vi "Measurement Logic.vi"() -> ()   [LabVIEW 2021, in "Efficiency And Load Regulation with Pin Map.lvlib"]
uses:
  Efficiency And Load Regulation with Pin Map.lvlib
  Measurement Configuration.ctl
  <instrlib>/niScope/Controls/niScope vertical coupling.ctl
  <instrlib>/niDMM/nidmm.llb/niDMM Resolution in Digits.ctl
  Measurement Results.ctl
  <vilib>/Plug-In SDKs/Measurements/Measure Call Context/Measure Call Context.lvclass
  subVIs/Reference values.ctl
  <vilib>/Plug-In SDKs/Clients/Session Management V1/Session Reservation/Session Reservation.lvclass
  common/Instrument Control/Scope/TClk/Instrument Info.ctl
  common/Instrument Control/Scope Parameters.ctl
  <instrlib>/niDMM/nidmm.llb/niDMM Trigger.ctl
  <instrlib>/niDMM/nidmm.llb/niDMM Sample Trigger.ctl
  subVIs/Additional measurements.ctl
  common/Instrument Control/DCPower Parameters.ctl
  <vilib>/Plug-In SDKs/Measurements/Measure Call Context/Reserve Sessions - NPin.vi
  <vilib>/Plug-In SDKs/Sessions/niDCPower/Initialize Sessions - NSess.vi
  <vilib>/Plug-In SDKs/Sessions/niDCPower/Get Connections - NPin MConn.vi
  <vilib>/Plug-In SDKs/Sessions/niDCPower/Get Connections - 1Pin 1Conn.vi
  <vilib>/Plug-In SDKs/Sessions/niScope/Initialize Sessions - NSess.vi
  <vilib>/Plug-In SDKs/Sessions/niScope/Get Connections - NPin MConn.vi
  <instrlib>/niScope/Configure/Trigger/niScope Configure Trigger Digital.vi
  <vilib>/Plug-In SDKs/Sessions/niDMM/Initialize Sessions - NSess.vi
  <vilib>/Plug-In SDKs/Sessions/niDMM/Get Connections - NPin MConn.vi
  <vilib>/Plug-In SDKs/Sessions/niDCPower/NI Session Management niDCPower.lvlib
  <vilib>/Plug-In SDKs/Sessions/niScope/NI Session Management niScope.lvlib
  common/PMIC Common.lvlib
  <vilib>/Plug-In SDKs/Sessions/niDMM/NI Session Management niDMM.lvlib
panel:
  out "measure call context out":refnum<class "Measure Call Context.lvclass">
  in  "measure call context in":refnum<class "Measure Call Context.lvclass">
  out "measurement results":T1
  in  "measurement configuration":T2={"Mode of operation"=enum."Perform measurement", "DUT setup time"=1.0, "Source delay"=0.005, "Aperture time"=0.005, "Nominal output voltage"=3.3, "Source pin name array"=[], "Source pin name index for efficiency"=0, "Source sense array"=[], "Source current limit array"=[], "Source maximum power array"=[], "Source start voltage array"=[], "Source stop voltage array"=[], "Source voltage sweep points"=10, "Use Source voltage array"=FALSE, "Source voltage concatenated array"=[], "Source voltage array size"=[], "Load pin name"="", "Load sense"=1009, "Load voltage limit range"=6.0, "Load sweep type"="Logarithmic", "Load start current"=0.1, "Load stop current"=24.0, "Load current sweep points/points per decade"=10, "Use Load current array"=FALSE, "Load current array"=[], "Pin Names for Scope"=[], "vertical range"=[], "vertical offset"=[], "probe attenuation"=[], "vertical coupling"=[], "channel enabled"=[], "input impedance"=[], "max input frequency"=[], "min sample rate"=[], "reference position"=[], "min record length"=[], "enforce realtime"=[], "dmm pin names"=[], "dmm function array"=[], "dmm resolution in digits array"=[], "dmm range array"=[]} {"dmm function array" items=["DC Volts", "AC Volts", "DC Current", "AC Current", "2-wire Resistance", "4-wire Resistance", "Diode", "Frequency", "Period", "AC Volts DC Coupled", "Capacitance", "Inductance", "Temperature"]; "Source sense array" items=["Local"=1008, "Remote"=1009]; "dmm resolution in digits array" items=["3 1/2"=3.5, "4 1/2"=4.5, "5 1/2"=5.5, "6 1/2"=6.5, "7 1/2"=7.5]; "input impedance" items=["1 mega ohm"=0, "50 ohms"=2]; "vertical coupling" items=["AC", "DC", "Ground"]; "Load sense" items=["Local"=1008, "Remote"=1009]}
  out "error out":errorcluster
  in  "error in":errorcluster
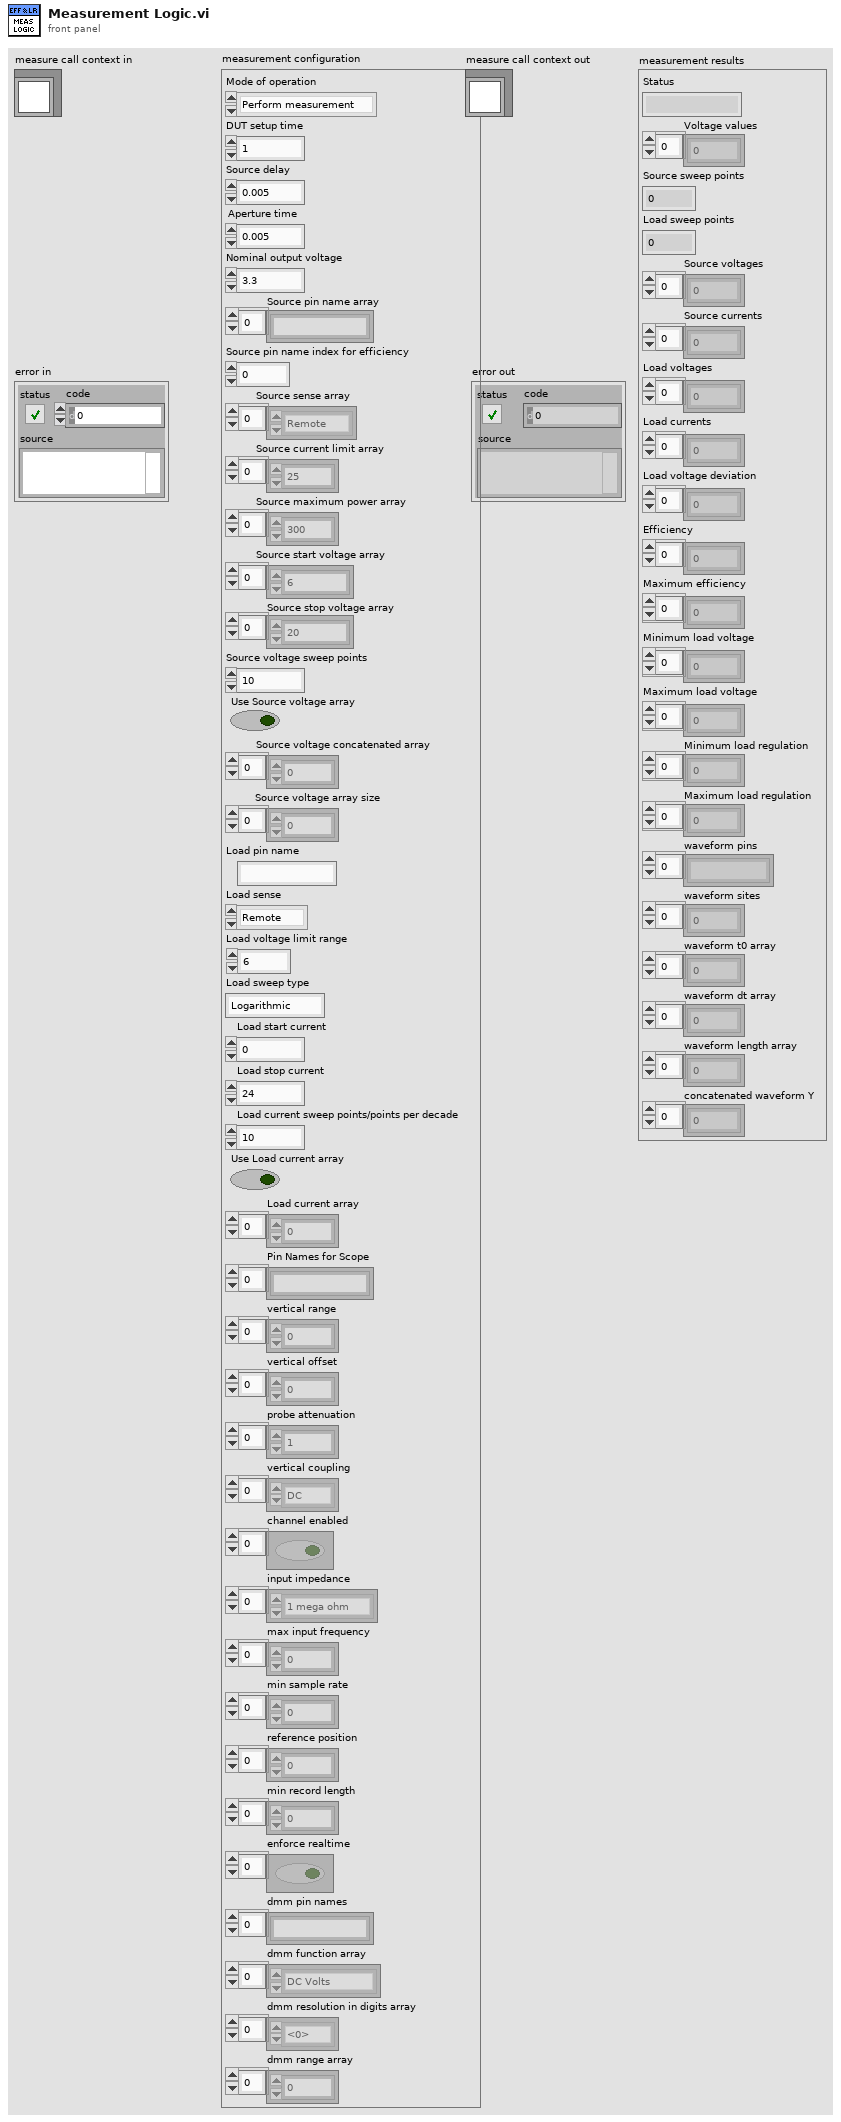
[diagram p1: front panel]
types:
  T1 = typedef "Efficiency And Load Regulation with Pin Map.lvlib/Measurement Results.ctl" = cluster{"Status":string, "Voltage values":dbl[], "Source sweep points":i32, "Load sweep points":i32, "Source voltages":dbl[], "Source currents":dbl[], "Load voltages":dbl[], "Load currents":dbl[], "Load voltage deviation":dbl[], "Efficiency":dbl[], "Maximum efficiency":dbl[], "Minimum load voltage":dbl[], "Maximum load voltage":dbl[], "Minimum load regulation":dbl[], "Maximum load regulation":dbl[], "waveform pins":string[], "waveform sites":i32[], "waveform t0 array":dbl[], "waveform dt array":dbl[], "waveform length array":i32[], "concatenated waveform Y":dbl[]}
  T2 = typedef "Efficiency And Load Regulation with Pin Map.lvlib/Measurement Configuration.ctl" = cluster{"Mode of operation":enum32{"Power on the DUT", "Perform measurement", "Power off the DUT"}, "DUT setup time":dbl, "Source delay":dbl, "Aperture time":dbl, "Nominal output voltage":dbl, "Source pin name array":string[], "Source pin name index for efficiency":i32, "Source sense array":i32[], "Source current limit array":dbl[], "Source maximum power array":dbl[], "Source start voltage array":dbl[], "Source stop voltage array":dbl[], "Source voltage sweep points":i32, "Use Source voltage array":bool, "Source voltage concatenated array":dbl[], "Source voltage array size":i32[], "Load pin name":string, "Load sense":i32, "Load voltage limit range":dbl, "Load sweep type":string, "Load start current":dbl, "Load stop current":dbl, "Load current sweep points/points per decade":i32, "Use Load current array":bool, "Load current array":dbl[], "Pin Names for Scope":string[], "vertical range":dbl[], "vertical offset":dbl[], "probe attenuation":dbl[], "vertical coupling":T3[], "channel enabled":bool[], "input impedance":u32[], "max input frequency":dbl[], "min sample rate":dbl[], "reference position":dbl[], "min record length":i32[], "enforce realtime":bool[], "dmm pin names":string[], "dmm function array":u32[], "dmm resolution in digits array":T4[], "dmm range array":dbl[]}
  T3 = typedef "niScope vertical coupling.ctl" = i32
  T4 = typedef "niDMM Resolution in Digits.ctl" = dbl
  T5 = typedef "Efficiency And Load Regulation with Pin Map.lvlib/Reference values.ctl" = cluster{"dcpower session reservation":refnum<class "Session Reservation.lvclass">, "Source handle array":refnum<k15>[], "Source channel name array":string[], "Load handle":refnum<k15>, "Load channel name":string, "Source voltage values":dbl[][], "Load current values":dbl[], "Number of steps":i32, "Source sequence name":string, "Source terminal name":string, "Measure terminal name":string, "scope session reservation":refnum<class "Session Reservation.lvclass">, "Scope handles":refnum<k15>[][], "connection map":map{string, T6[]}, "instrument info map array":map{string, cluster{"channel":string, "siteNumber":i32, "pin":string, "Scope Parameters":T7}[]}[], "Enable TClk":bool, "dmm session reservation":refnum<class "Session Reservation.lvclass">, "dmm handle array":refnum<k15>[], "DMM Trigger Source":T8, "DMM Sample Trigger":T9, "Measurement Results":T1, "Additional measurements":T10}
  T6 = typedef "PMIC Common.lvlib/Instrument Info.ctl" = cluster{"instrument":string, "channel":string, "siteNumber":i32}
  T7 = typedef "PMIC Common.lvlib/Scope Parameters.ctl" = cluster{"vertical range":dbl, "vertical offset":dbl, "probe attenuation":dbl, "vertical coupling":T3, "channel enabled":bool, "input impedance":u32, "maximum input frequency":dbl, "min sample rate":dbl, "reference position":dbl, "min record length":i32, "number of records":i32, "enforce realtime":bool}
  T8 = typedef "niDMM Trigger.ctl" = enum16{"Immediate", "External", "TTL 0", "TTL 1", "TTL 2", "TTL 3", "TTL 4", "TTL 5", "TTL 6", "Software", "TTL 7", "PXI Star", "LBR Trig 1", "Aux Trig 1"}
  T9 = typedef "niDMM Sample Trigger.ctl" = enum16{"Immediate", "External", "TTL 0", "TTL 1", "TTL 2", "TTL 3", "TTL 4", "TTL 5", "TTL 6", "Interval", "Software", "TTL 7", "PXI Star", "LBR Trig 1", "Aux Trig 1"}
  T10 = typedef "Efficiency And Load Regulation with Pin Map.lvlib/Additional measurements.ctl" = cluster{"voltage measurements from all sources":dbl[][], "current measurements from all sources":dbl[][], "all dmm measurements":dbl[][], "all scope waverforms":waveform(dbl)[]}
  T11 = enum32{"Power on the DUT", "Perform measurement", "Power off the DUT"}
  T12 = typedef "PMIC Common.lvlib/DCPower Parameters.ctl" = cluster{"Supply":dbl, "Limit":dbl, "Aperture Time":dbl, "Settling Time":dbl, "Sense":i32, "Transient Response":i32}
  T13 = enum16{"PXI_Trig0", "PXI_Trig1", "PXI_Trig2", "PXI_Trig3", "PXI_Trig4", "PXI_Trig5", "PXI_Trig6", "PXI_Trig7"}
  T14 = typedef "NI Session Management niDCPower.lvlib/Connection with Session.ctl" = cluster{"connection":T15, "session":refnum<k15>}
  T15 = typedef "NI Session Management V1 Client.lvlib/Session Reservation.lvclass/Connection.ctl" = cluster{"pin or relay name":string, "site":i32, "instrument type id":string, "channel":string}
  T16 = typedef "PMIC Common.lvlib/DCPower Parameters for Adv Sequence.ctl" = cluster{"Supplies":dbl[], "Limits":dbl[], "Aperture Time":dbl, "Settling Time":dbl, "Sense":i32, "Transient Response":i32}
  T17 = typedef "PMIC Common.lvlib/DCPower Parameters for Sequence.ctl" = cluster{"Supplies":dbl[], "Limit":dbl, "Aperture Time":dbl, "Settling Time":dbl, "Sense":i32, "Transient Response":i32}
  T18 = typedef "NI Session Management niScope.lvlib/Connection with Session.ctl" = cluster{"connection":T15, "session":refnum<k15>}
  T19 = typedef "NI Measurement Plug-In SDK.lvlib/Pin Map Context.ctl" = cluster{"pin map id":string, "sites":i32[]}
  T20 = map{string, cluster{"channel":string, "siteNumber":i32, "pin":string, "Scope Parameters":T7}[]}[]
  T21 = typedef "NI Session Management niDMM.lvlib/Connection with Session.ctl" = cluster{"connection":T15, "session":refnum<k15>}
  T22 = typedef "PMIC Common.lvlib/DMM Parameters.ctl" = cluster{"Function":T23, "Resolution in Digits":T4, "Range":dbl, "Trigger Source":T8, "Trigger Delay (sec)":dbl, "Trigger Count":i32, "Sample Count":i32, "Sample Trigger":T9, "Sample Interval (sec)":dbl, "Trigger Slope":T24, "Sample Trigger Slope":T24}
  T23 = typedef "niDMM Function.ctl" = enum16{"DC Volts", "AC Volts", "DC Current", "AC Current", "2-wire Resistance", "4-wire Resistance", "Diode", "Frequency", "Period", "AC Volts DC Coupled", "Capacitance", "Inductance", "Temperature"}
  T24 = typedef "niDMM Slope.ctl" = enum16{"Rising Edge", "Falling Edge"}
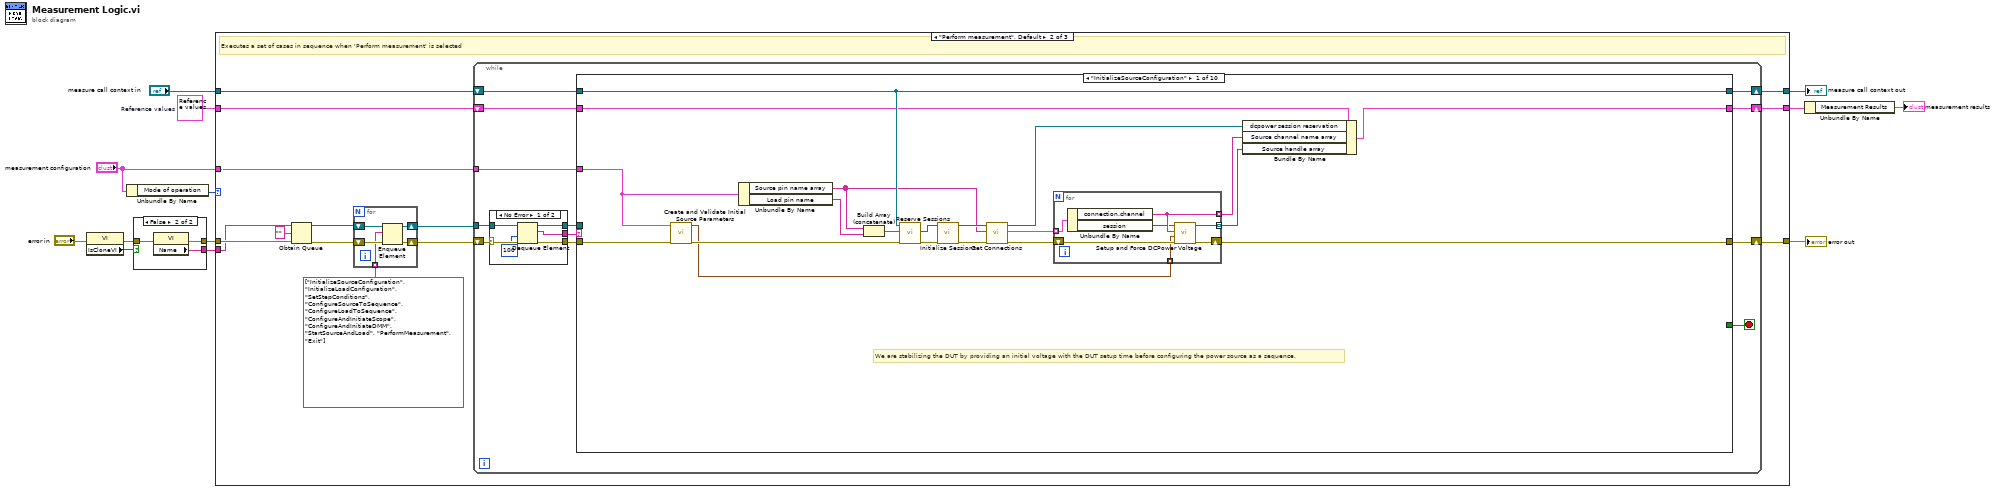
[diagram p0: block diagram]
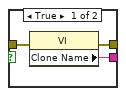
[diagram p2: hidden frame]
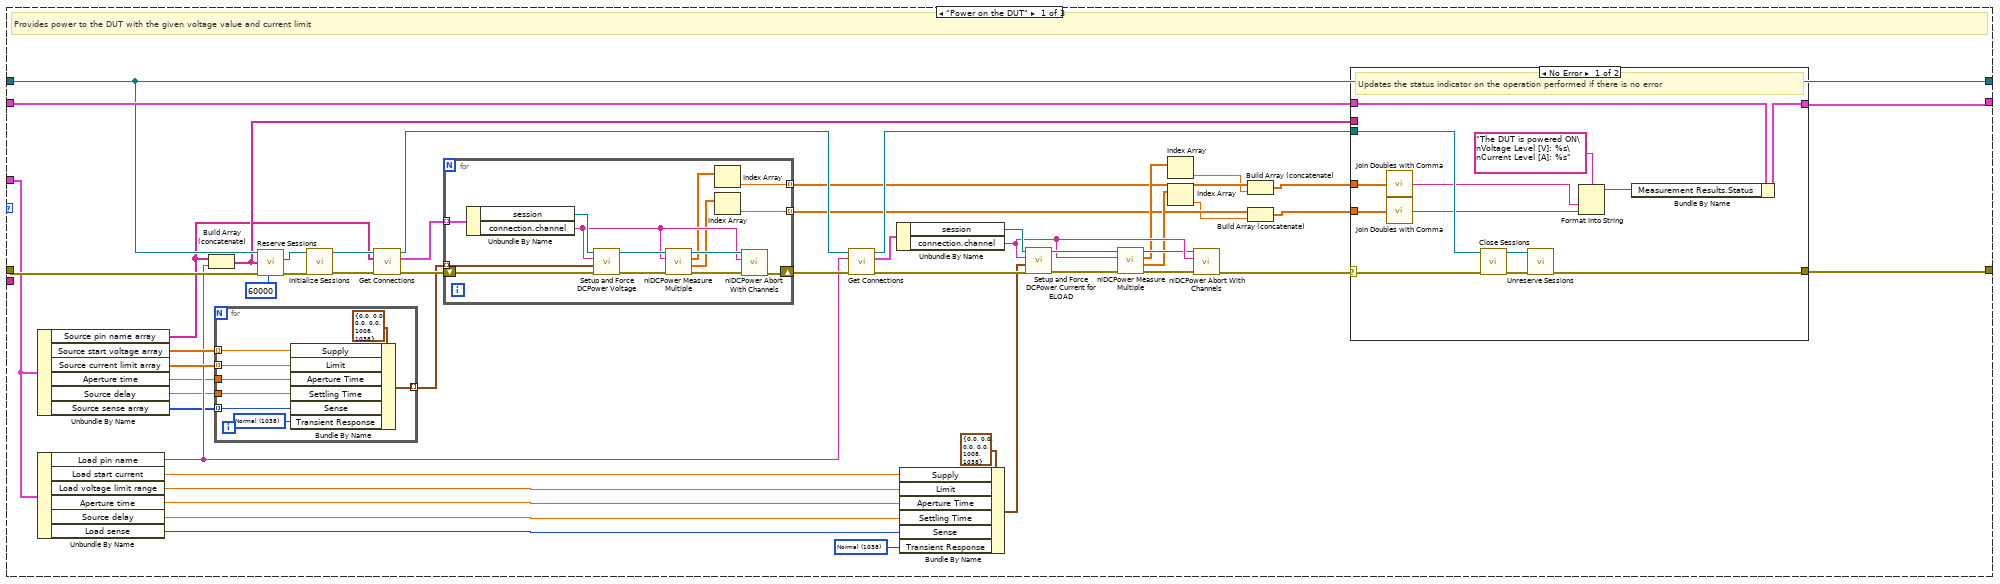
[diagram p3: hidden frame]
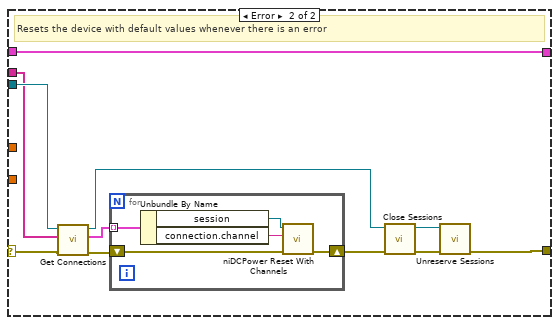
[diagram p4: hidden frame]
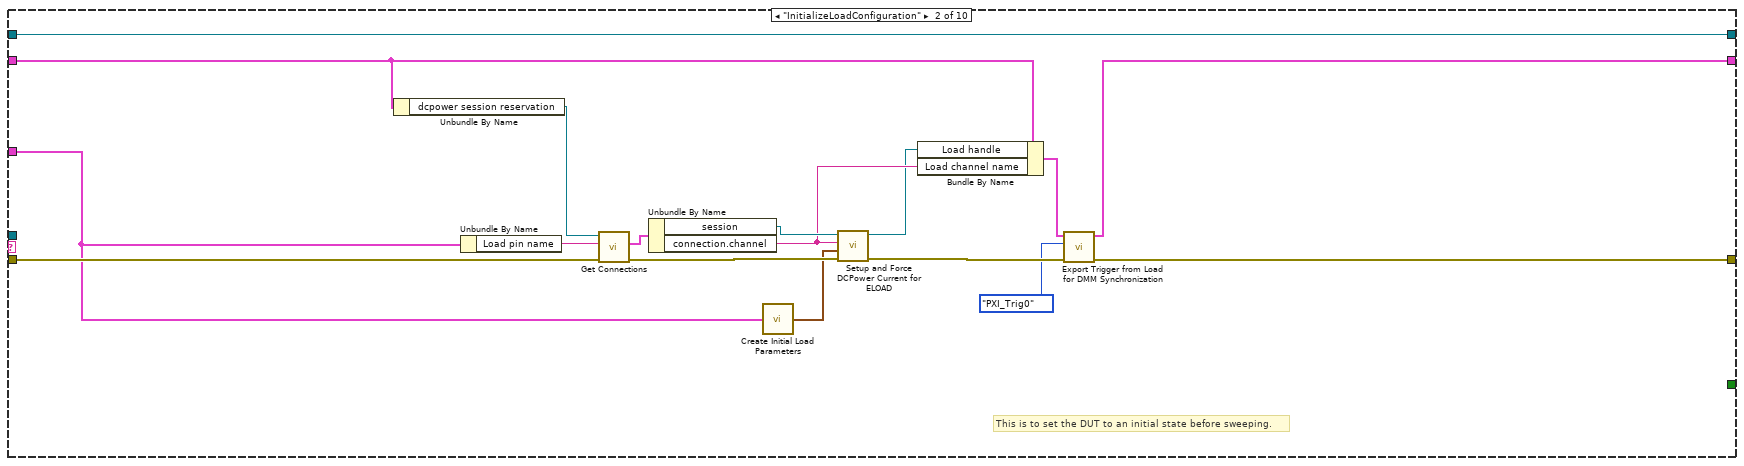
[diagram p5: hidden frame]
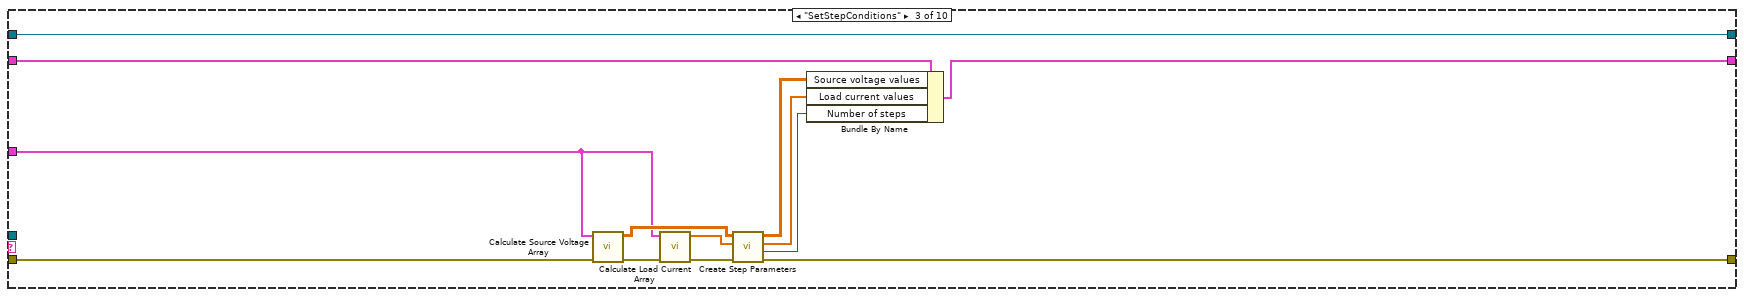
[diagram p6: hidden frame]
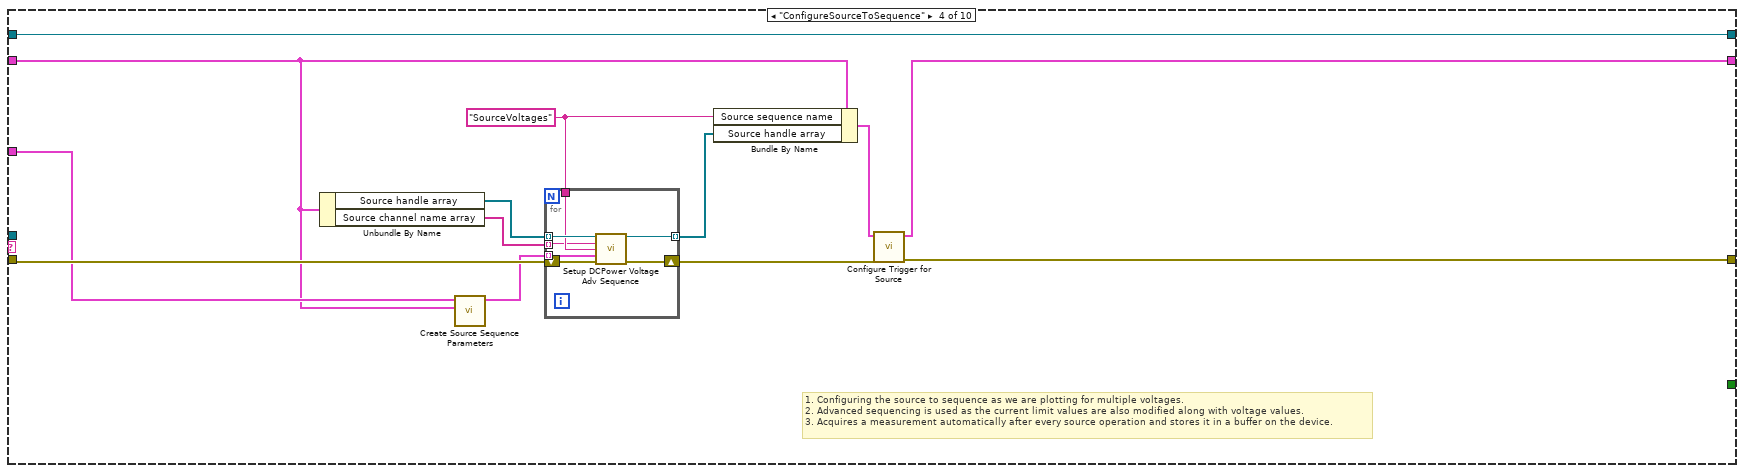
[diagram p7: hidden frame]
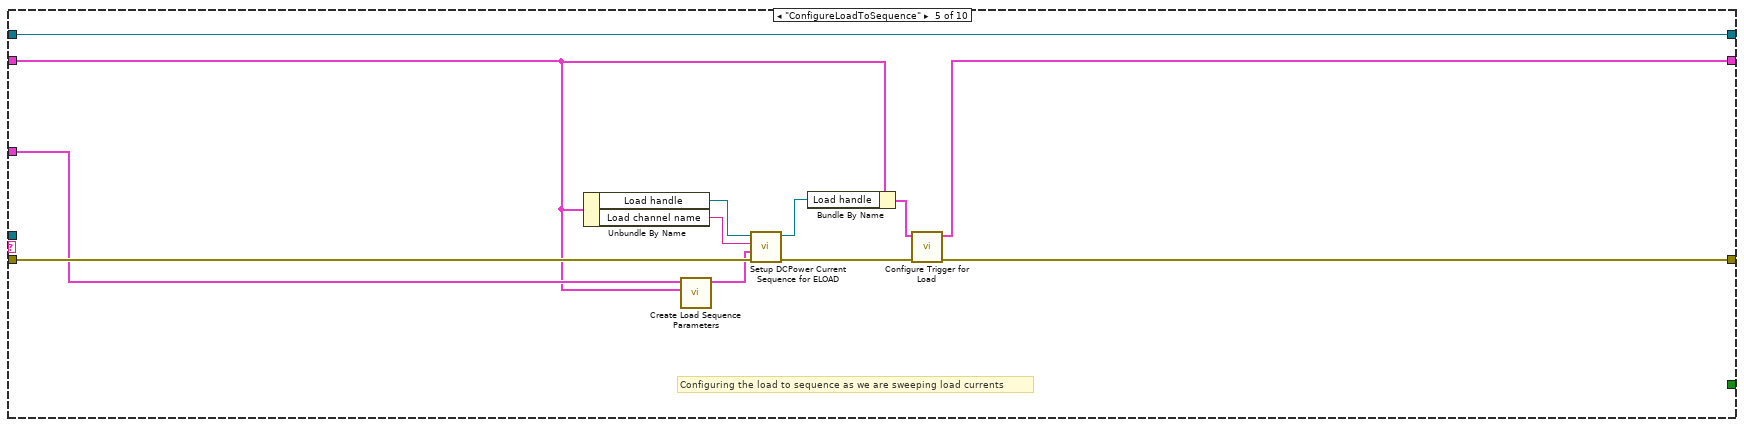
[diagram p8: hidden frame]
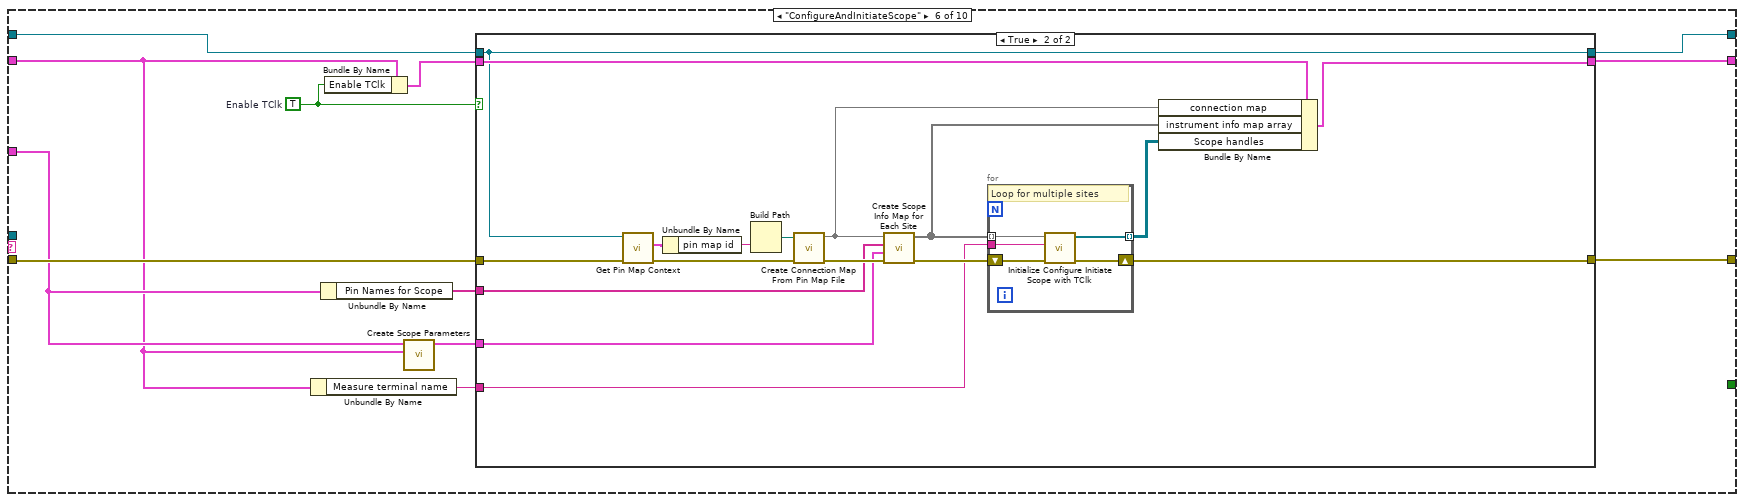
[diagram p9: hidden frame]
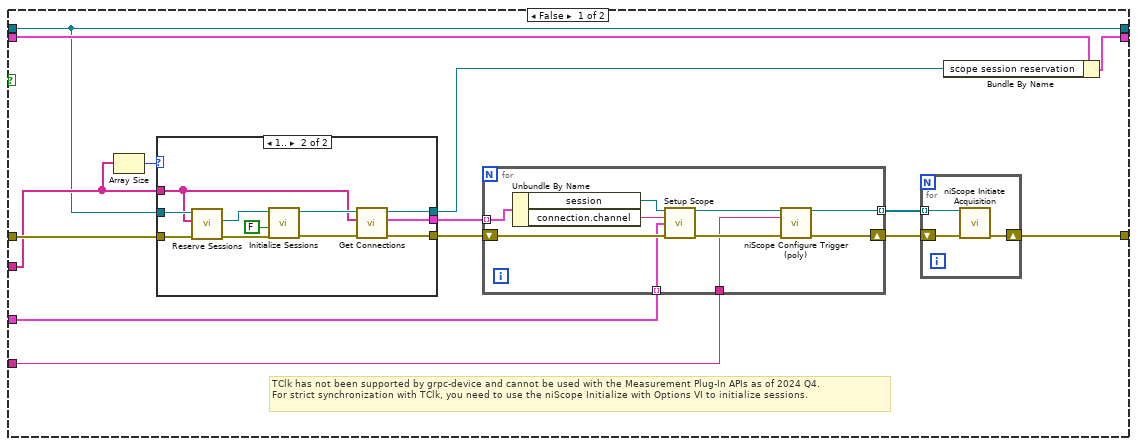
[diagram p10: hidden frame]
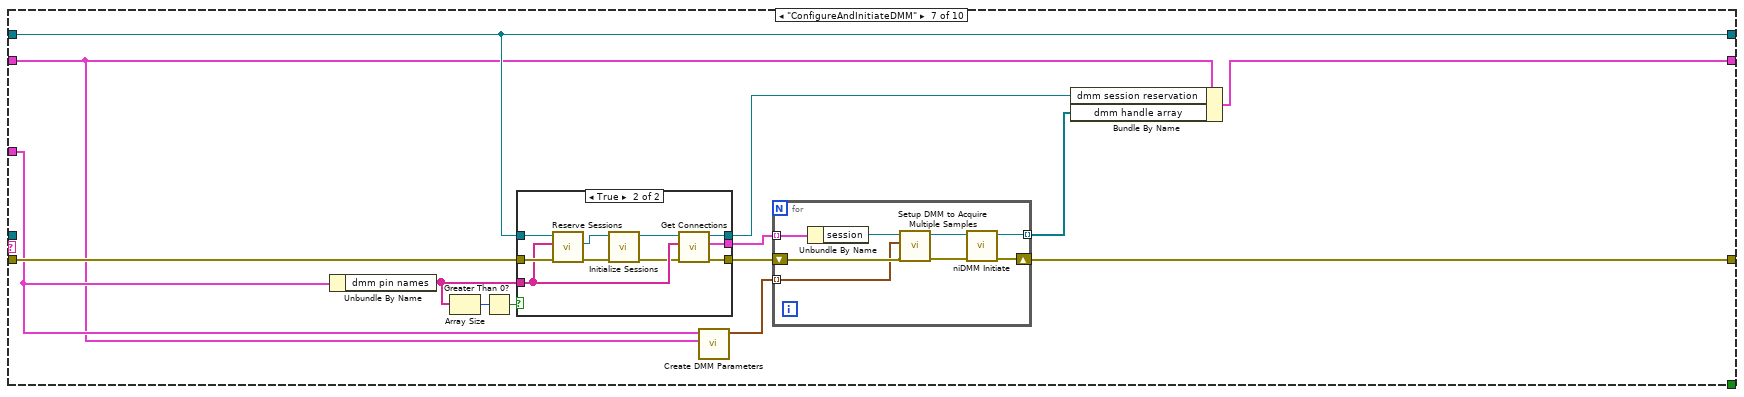
[diagram p12: hidden frame]
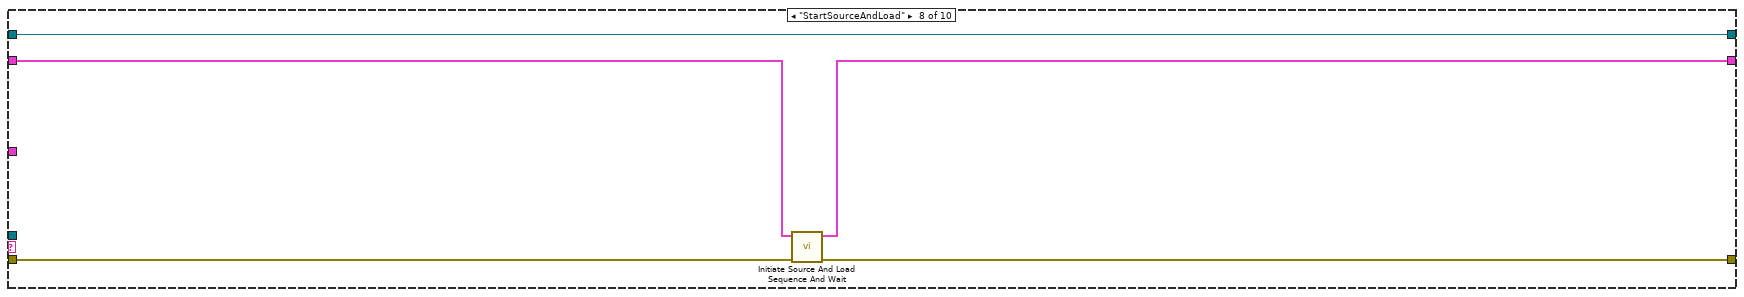
[diagram p14: hidden frame]
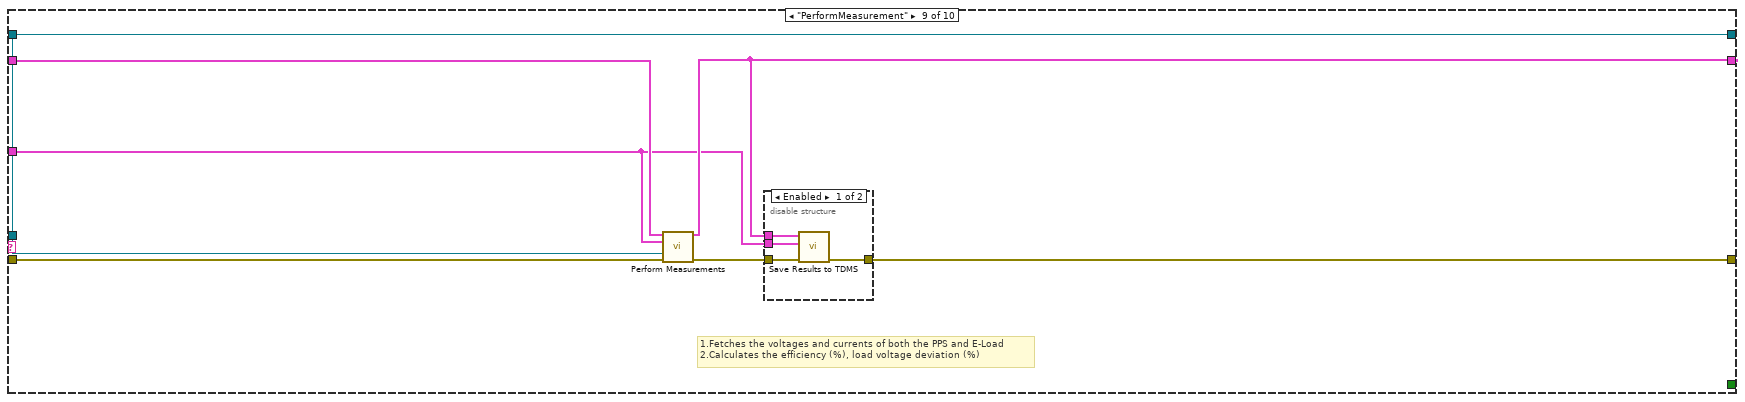
[diagram p15: hidden frame]
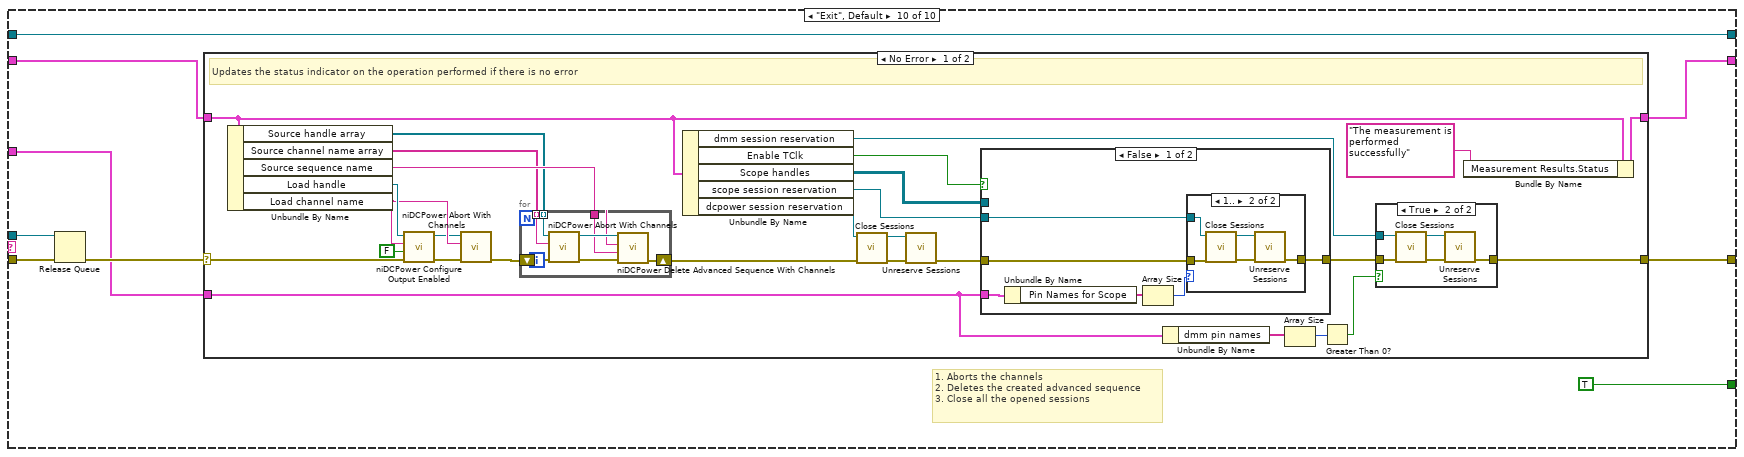
[diagram p17: hidden frame]
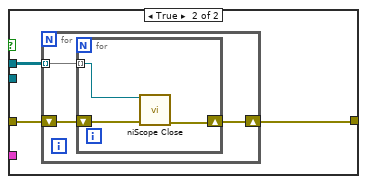
[diagram p20: hidden frame]
diagram:
  w12 = T5 {"dcpower session reservation"=refnum, "Source handle array"=[], "Source channel name array"=[], "Load handle"="", "Load channel name"="", "Source voltage values"=[], "Load current values"=[], "Number of steps"=0, "Source sequence name"="", "Source terminal name"="", "Measure terminal name"="", "scope session reservation"=refnum, "Scope handles"=[], "connection map"={}, "instrument info map array"=[], "Enable TClk"=FALSE, "dmm session reservation"=refnum, "dmm handle array"=[], "DMM Trigger Source"=enum."Immediate", "DMM Sample Trigger"=enum."TTL 0", "Measurement Results"={"Status"="", "Voltage values"=[], "Source sweep points"=0, "Load sweep points"=0, "Source voltages"=[], "Source currents"=[], "Load voltages"=[], "Load currents"=[], "Load voltage deviation"=[], "Efficiency"=[], "Maximum efficiency"=[], "Minimum load voltage"=[], "Maximum load voltage"=[], "Minimum load regulation"=[], "Maximum load regulation"=[], "waveform pins"=[], "waveform sites"=[], "waveform t0 array"=[], "waveform dt array"=[], "waveform length array"=[], "concatenated waveform Y"=[]}, "Additional measurements"={"voltage measurements from all sources"=[], "current measurements from all sources"=[], "all dmm measurements"=[], "all scope waverforms"=[]}}  # Reference values
  n1 = property class="VI"(error in="error in") -> (error out=w4:errorcluster, "IsCloneVI"=w5:bool)  [unwired: 1 in, 1 out]
  n2 = Unbundle By Name("measurement configuration") -> ("Mode of operation"=w10:T11)
  n3 = case shown="False" w5 {
    tunnel: [w16 w19] -> w2
    tunnel: [w15 w18] -> w1
    tunnel: w4 -> [w14 w17]
    frame True {
      n4 = property class="VI"(error in=w14) -> (error out=w16:errorcluster, "Clone Name"=w15:string)  [unwired: 1 in, 1 out]
    }
    frame False {
      n5 = property class="VI"(error in=w17) -> (error out=w19:errorcluster, "Name"=w18:string)  [unwired: 1 in, 1 out]
    }
  }
  n6 = case shown="\"Perform measurement\", Default" w10 {
    tunnel: [w67 w122 w502] -> w6
    tunnel: w2 -> [w57 w123 w521]
    tunnel: "measurement configuration" -> [w31 w129 w530]
    tunnel: [w68 w124 w527] -> w7
    tunnel: w12 -> [w69 w128 w529]
    tunnel: "measure call context in" -> [w58 w126 w519]
    tunnel: [w58 w125 w519] -> w8
    tunnel: w1 -> [_ w121 _]
    frame "Power on the DUT" {
      w22 = 1038 items=["Slow"=1041, "Normal"=1038, "Fast"=1039, "Custom"=1042] ("Transient Response")
      # "Provides power to the DUT with the given voltage value and current limit"
      n7 = Unbundle By Name(w31) -> ("Source pin name array"=w32:string[], "Source start voltage array"=w60:dbl[], "Source current limit array"=w59:dbl[], "Aperture time"=w28:dbl, "Source delay"=w27:dbl, "Source sense array"=w26:i32[])
      n8 = Unbundle By Name(w31) -> ("Load pin name"=w30:string, "Load start current"=w25:dbl, "Load voltage limit range"=w24:dbl, "Aperture time"=w21:dbl, "Source delay"=w20:dbl, "Load sense"=w23:i32)
      n9 = Build Array (concatenate)(w32, w30) -> (w33:string[])
      n10 = for {
        tunnel: w60 -> [w77] mode=indexing
        tunnel: w59 -> [w76] mode=indexing
        tunnel: [w74] -> w29 mode=indexing
        tunnel: w28 -> [w73]
        tunnel: w27 -> [w71]
        tunnel: w26 -> [w72] mode=indexing
        w70 = 1038 items=["Slow"=1041, "Normal"=1038, "Fast"=1039, "Custom"=1042] ("Transient Response")
        n11 = Bundle By Name(cluster=T12 {"Supply"=0.0, "Limit"=0.0, "Aperture Time"=0.0, "Settling Time"=0.0, "Sense"=1008, "Transient Response"=1038} ("DCPower Parameters"), "Supply"=w77, "Limit"=w76, "Aperture Time"=w73, "Settling Time"=w71, "Sense"=w72, "Transient Response"=w70) -> (w74:T12)
      }
      n12 = call-poly <vilib>:"Reserve Sessions.vi"("timeout (ms)"=60000, "error in"=w57, "pin or relay names"=w33, "measurement context in"=w58) -> ("error out"=w66:errorcluster, "session reservation out"=w65:refnum<class "Session Reservation.lvclass">)  [unwired: 5 in, 1 out]
      n13 = call-poly <vilib>:"Initialize Sessions.vi"("error in"=w66, "session reservation in"=w65) -> ("error out"=w64:errorcluster, "session reservation out"=w63:refnum<class "Session Reservation.lvclass">)  [unwired: 6 in, 2 out]
      n14 = call-poly <vilib>:"Get Connections.vi"("error in"=w64, "pin or relay names"=w32, "session reservation in"=w63) -> ("error out"=w61:errorcluster, "connections"=w56:T14[], "session reservation out"=w53:refnum<class "Session Reservation.lvclass">)  [unwired: 6 in]
      n15 = for {
        tunnel: w56 -> [w90] mode=indexing
        tunnel: w29 -> [w88] mode=indexing
        shift-right: [w85] -> w55
        shift-left: w61 -> [w91]
        tunnel: [w79] -> w39 mode=indexing
        tunnel: [w78] -> w36 mode=indexing
        n16 = Unbundle By Name(w90) -> ("session"=w89:refnum<k15>, "connection.channel"=w82:string)
        n17 = call "Setup and Force DCPower Voltage.vi"("error in"=w91, "Parameters"=w88, "Channel List"=w82, "DCPower Handle In"=w89) -> ("error out"=w87:errorcluster, "DCPower Handle Out"=w86:refnum<k15>)  [unwired: 6 in]
        n18 = call <instrlib>:"niDCPower Measure Multiple.vi"("error in (no error)"=w87, "channel name"=w82, "instrument handle"=w86) -> ("error out"=w84:errorcluster, "current measurements"=w80:dbl[], "voltage measurements"=w81:dbl[], "instrument handle out"=w83:refnum<k15>)  [unwired: 5 in]
        n19 = Index Array(array=w81) -> (element=w79:dbl)  [unwired: 1 in]
        n20 = Index Array(array=w80) -> (element=w78:dbl)  [unwired: 1 in]
        n21 = call <instrlib>:"niDCPower Abort With Channels.vi"("error in (no error)"=w84, "channel name"=w82, "instrument handle"=w83) -> ("error out"=w85:errorcluster)  [unwired: 7 in, 1 out]
      }
      n22 = call-poly <vilib>:"Get Connections.vi"("error in"=w55, "pin or relay name"=w30, "session reservation in"=w53) -> ("error out"=w50:errorcluster, "connection"=w54:T14, "session reservation out"=w52:refnum<class "Session Reservation.lvclass">)  [unwired: 6 in]
      n23 = Unbundle By Name(w54) -> ("session"=w51:refnum<k15>, "connection.channel"=w43:string)
      n24 = Bundle By Name(cluster=T12 {"Supply"=0.0, "Limit"=0.0, "Aperture Time"=0.0, "Settling Time"=0.0, "Sense"=1008, "Transient Response"=1038} ("DCPower Parameters"), "Supply"=w25, "Limit"=w24, "Aperture Time"=w21, "Settling Time"=w20, "Sense"=w23, "Transient Response"=w22) -> (w48:T12)
      n25 = call "Setup and Force DCPower Current for ELOAD.vi"("error in"=w50, "Parameters"=w48, "Channel List"=w43, "DCPower Handle In"=w51) -> ("error out"=w46:errorcluster, "DCPower Handle Out"=w44:refnum<k15>)  [unwired: 6 in]
      n26 = call <instrlib>:"niDCPower Measure Multiple.vi"("error in (no error)"=w46, "channel name"=w43, "instrument handle"=w44) -> ("error out"=w47:errorcluster, "current measurements"=w40:dbl[], "voltage measurements"=w41:dbl[], "instrument handle out"=w42:refnum<k15>)  [unwired: 5 in]
      n27 = Index Array(array=w41) -> (element=w38:dbl)  [unwired: 1 in]
      n28 = Index Array(array=w40) -> (element=w35:dbl)  [unwired: 1 in]
      n29 = call <instrlib>:"niDCPower Abort With Channels.vi"("error in (no error)"=w47, "channel name"=w43, "instrument handle"=w42) -> ("error out"=w45:errorcluster)  [unwired: 7 in, 1 out]
      n30 = Build Array (concatenate)(w39, w38) -> (w37:dbl[])
      n31 = Build Array (concatenate)(w36, w35) -> (w34:dbl[])
      n32 = case shown="No Error" w45 {
        selector: w45 -> [w99 w110]
        tunnel: [w98 w111] -> w67
        tunnel: [w104 w115] -> w68
        tunnel: w69 -> [w101 w115]
        tunnel: w52 -> [w97 w107]
        tunnel: w37 -> [w95 _]
        tunnel: w34 -> [w94 _]
        tunnel: w33 -> [_ w105]
        frame No Error {
          # "Updates the status indicator on the operation performed if there is no error"
          n33 = call "Join Doubles with Comma.vi"("double array"=w95) -> ("joined string"=w93:string)
          n34 = call "Join Doubles with Comma.vi"("double array"=w94) -> ("joined string"=w92:string)
          n35 = call <vilib>:"Close Sessions.vi"("error in"=w99, "session reservation in"=w97) -> ("error out"=w100:errorcluster, "session reservation out"=w96:refnum<class "Session Reservation.lvclass">)  [unwired: 8 in]
          n36 = call <vilib>:"Unreserve Sessions.vi"("error in"=w100, "session reservation in"=w96) -> ("error out"=w98:errorcluster)  [unwired: 9 in]
          n37 = Format Into String(format string="The DUT is powered ON\nVoltage Level [V]: %s\nCurrent Level [A]: %s" ("message"), w93, w92) -> (resulting string=w102:string)  [unwired: 2 in, 1 out]
          n38 = Bundle By Name(cluster=w101, "Measurement Results.Status"=w102) -> (w104:T5)
        }
        frame Error {
          # "Resets the device with default values whenever there is an error"
          n39 = call-poly <vilib>:"Get Connections.vi"("error in"=w110, "pin or relay names"=w105, "session reservation in"=w107) -> ("error out"=w109:errorcluster, "connections"=w108:T14[], "session reservation out"=w106:refnum<class "Session Reservation.lvclass">)  [unwired: 6 in]
          n40 = for {
            shift-right: [w119] -> w112
            shift-left: w109 -> [w120]
            tunnel: w108 -> [w116] mode=indexing
            n41 = Unbundle By Name(w116) -> ("session"=w118:refnum<k15>, "connection.channel"=w117:string)
            n42 = call <instrlib>:"niDCPower Reset With Channels.vi"("error in (no error)"=w120, "channel name"=w117, "instrument handle"=w118) -> ("error out"=w119:errorcluster)  [unwired: 7 in, 1 out]
          }
          n43 = call <vilib>:"Close Sessions.vi"("error in"=w112, "session reservation in"=w106) -> ("error out"=w114:errorcluster, "session reservation out"=w113:refnum<class "Session Reservation.lvclass">)  [unwired: 8 in]
          n44 = call <vilib>:"Unreserve Sessions.vi"("error in"=w114, "session reservation in"=w113) -> ("error out"=w111:errorcluster)  [unwired: 9 in]
        }
      }
    }
    frame "Perform measurement", Default {
      # "Executes a set of cases in sequence when 'Perform measurement' is selected"
      n45 = Obtain Queue(name (unnamed)=w121, element data type="", error in (no error)=w123) -> (queue out=w133:refnum<queue>, error out=w134:errorcluster)  [unwired: 2 in, 1 out]
      n46 = for {
        shift-right: [w498] -> w130
        shift-left: w133 -> [w500]
        shift-right: [w497] -> w127
        shift-left: w134 -> [w499]
        tunnel: string[] ["InitializeSourceConfiguration", "InitializeLoadConfiguration", "SetStepConditions", "ConfigureSourceToSequence", "ConfigureLoadToSequence", "ConfigureAndInitiateScope", "ConfigureAndInitiateDMM", "StartSourceAndLoad", "PerformMeasurement", "Exit"] ("Step sequence") -> [w496] mode=indexing
        n47 = Enqueue Element(queue=w500, element=w496, error in (no error)=w499) -> (queue out=w498:refnum<queue>, error out=w497:errorcluster)  [unwired: 1 in, 1 out]
      }
      n48 = while {
        tunnel: w130 -> [w146]
        tunnel: w129 -> [w142]
        shift-right: [w139] -> w124
        shift-left: w128 -> [w140]
        shift-right: [w138] -> w122
        shift-left: w127 -> [w145]
        shift-right: [w135] -> w125
        shift-left: w126 -> [w137]
        stop <- w136 stop-if-true
        n49 = case shown="No Error" w145 {
          selector: w145 -> [w490 w494]
          tunnel: w146 -> [w492 w493]
          tunnel: [w491 "Exit" ("t")] -> w144
          tunnel: [w489 w494] -> w141
          tunnel: [w487 w493] -> w143
          frame No Error {
            n50 = Dequeue Element(queue=w492, timeout in ms (-1)=100, error in (no error)=w490) -> (queue out=w487:refnum<queue>, element=w491:string, error out=w489:errorcluster)  [unwired: 1 out]
          }
          frame Error {
          }
        }
        n51 = case shown="\"InitializeSourceConfiguration\"" w144 {
          tunnel: w143 -> [_ _ _ _ _ _ _ _ _ w362]
          tunnel: w142 -> [w149 w181 w192 w208 w229 w238 w314 _ w347 w360]
          tunnel: w141 -> [w148 w190 w201 w214 w232 w247 w322 w345 w353 w367]
          tunnel: w140 -> [w152 w188 w202 w206 w226 w237 w312 w343 w350 w365]
          tunnel: [w166 w175 w203 w209 w234 w246 w315 w342 w348 w363] -> w139
          tunnel: [w154 w178 w196 w216 w235 w245 w318 w344 w349 w364] -> w138
          tunnel: w137 -> [w156 w183 w191 w211 w230 w240 w321 w346 w352 w359]
          tunnel: [_ _ _ _ _ _ _ _ _ TRUE] -> w136
          tunnel: [w156 w183 w191 w211 w230 w239 w321 w346 w352 w359] -> w135
          frame "InitializeSourceConfiguration" {
            # "We are stabilizing the DUT by providing an initial voltage with the DUT setup time before configuring the power source as a sequence."
            n52 = call "Create and Validate Initial Source Parameters.vi"("error in (no error)"=w148, "measurement configuration"=w149) -> ("error out"=w150:errorcluster, "Initial source parameters"=w147:T12[])  [unwired: 8 in]
            n53 = Unbundle By Name(w149) -> ("Source pin name array"=w155:string[], "Load pin name"=w160:string)
            n54 = Build Array (concatenate)(w155, w160) -> (w159:string[])
            n55 = call-poly <vilib>:"Reserve Sessions.vi"("error in"=w150, "pin or relay names"=w159, "measurement context in"=w156) -> ("error out"=w165:errorcluster, "session reservation out"=w164:refnum<class "Session Reservation.lvclass">)  [unwired: 6 in, 1 out]
            n56 = call-poly <vilib>:"Initialize Sessions.vi"("error in"=w165, "session reservation in"=w164) -> ("error out"=w163:errorcluster, "session reservation out"=w162:refnum<class "Session Reservation.lvclass">)  [unwired: 6 in, 2 out]
            n57 = call-poly <vilib>:"Get Connections.vi"("error in"=w163, "pin or relay names"=w155, "session reservation in"=w162) -> ("error out"=w151:errorcluster, "connections"=w161:T14[], "session reservation out"=w153:refnum<class "Session Reservation.lvclass">)  [unwired: 6 in]
            n58 = for {
              tunnel: w161 -> [w173] mode=indexing
              tunnel: [w172] -> w158 mode=indexing
              tunnel: [w169] -> w157 mode=indexing
              tunnel: w147 -> [w167] mode=indexing
              shift-right: [w168] -> w154
              shift-left: w151 -> [w170]
              n59 = Unbundle By Name(w173) -> ("connection.channel"=w172:string, "session"=w171:refnum<k15>)
              n60 = call "Setup and Force DCPower Voltage.vi"("error in"=w170, "Parameters"=w167, "Channel List"=w172, "DCPower Handle In"=w171) -> ("error out"=w168:errorcluster, "DCPower Handle Out"=w169:refnum<k15>)  [unwired: 6 in]
            }
            n61 = Bundle By Name(cluster=w152, "dcpower session reservation"=w153, "Source channel name array"=w158, "Source handle array"=w157) -> (w166:T5)
          }
          frame "InitializeLoadConfiguration" {
            # "This is to set the DUT to an initial state before sweeping."
            n62 = Unbundle By Name(w188) -> ("dcpower session reservation"=w187:refnum<class "Session Reservation.lvclass">)
            n63 = Unbundle By Name(w181) -> ("Load pin name"=w184:string)
            n64 = call-poly <vilib>:"Get Connections.vi"("error in"=w190, "pin or relay name"=w184, "session reservation in"=w187) -> ("error out"=w185:errorcluster, "connection"=w189:T14)  [unwired: 6 in, 1 out]
            n65 = Unbundle By Name(w189) -> ("session"=w186:refnum<k15>, "connection.channel"=w182:string)
            n66 = call "Create Initial Load Parameters.vi"("measurement configuration"=w181) -> ("initial load parameters"=w180:T12)
            n67 = call "Setup and Force DCPower Current for ELOAD.vi"("error in"=w185, "Parameters"=w180, "Channel List"=w182, "DCPower Handle In"=w186) -> ("error out"=w179:errorcluster, "DCPower Handle Out"=w177:refnum<k15>)  [unwired: 6 in]
            n68 = Bundle By Name(cluster=w188, "Load handle"=w177, "Load channel name"=w182) -> (w176:T5)
            n69 = call "Export Trigger from Load for DMM Synchronization.vi"("error in (no error)"=w179, "DMM Trigger Source"=T13."PXI_Trig0", "Reference values"=w176) -> ("error out"=w178:errorcluster, "Reference values out"=w175:T5)  [unwired: 7 in]
          }
          frame "SetStepConditions" {
            n70 = call "Calculate Source Voltage Array.vi"("error in"=w201, "measurement configuration"=w192) -> ("error out"=w200:errorcluster, "Source voltage array"=w197:dbl[][])  [unwired: 7 in, 1 out]
            n71 = call "Calculate Load Current Array.vi"("error in"=w200, "measurement configuration"=w192) -> ("error out"=w199:errorcluster, "Load current array"=w198:dbl[])  [unwired: 7 in, 1 out]
            n72 = call "Create Step Parameters.vi"("error in (no error)"=w199, "Load current array"=w198, "Source voltage array"=w197) -> ("error out"=w196:errorcluster, "Number of steps"=w193:i32, "Load current values"=w194:dbl[], "Source voltage values"=w195:dbl[][])  [unwired: 5 in]
            n73 = Bundle By Name(cluster=w202, "Source voltage values"=w195, "Load current values"=w194, "Number of steps"=w193) -> (w203:T5)
          }
          frame "ConfigureSourceToSequence" {
            w213 = "SourceVoltages" ("sequence name")
            # "1. Configuring the source to sequence as we are plotting for multiple voltages.\n2. Advanced sequencing is used as the current limit values are also modified along with voltage values.\n3. Acquires a measurement automatically after every source operation and stores it in a buffer on the device."
            n74 = Unbundle By Name(w206) -> ("Source handle array"=w215:refnum<k15>[], "Source channel name array"=w205:string[])
            n75 = call "Create Source Sequence Parameters.vi"("Reference values"=w206, "measurement configuration"=w208) -> ("source sequence parameters"=w207:T16[])  [unwired: 9 in]
            n76 = for {
              tunnel: w215 -> [w223] mode=indexing
              tunnel: w207 -> [w222] mode=indexing
              tunnel: w213 -> [w220]
              tunnel: [w219] -> w204 mode=indexing
              tunnel: w205 -> [w217] mode=indexing
              shift-right: [w218] -> w212
              shift-left: w214 -> [w221]
              n77 = call "Setup DCPower Voltage Adv Sequence.vi"("DCPower Handle In"=w223, "Channel List"=w217, "Sequence Name"=w220, "Parameters for Adv Sequence"=w222, "error in (no error)"=w221) -> ("DCPower Handle Out"=w219:refnum<k15>, "error out"=w218:errorcluster)  [unwired: 9 in]
            }
            n78 = Bundle By Name(cluster=w206, "Source sequence name"=w213, "Source handle array"=w204) -> (w210:T5)
            n79 = call "Configure Trigger for Source.vi"("error in (no error)"=w212, "Reference values"=w210) -> ("error out"=w216:errorcluster, "Reference values out"=w209:T5)  [unwired: 8 in]
          }
          frame "ConfigureLoadToSequence" {
            # "Configuring the load to sequence as we are sweeping load currents"
            n80 = Unbundle By Name(w226) -> ("Load handle"=w233:refnum<k15>, "Load channel name"=w228:string)
            n81 = call "Create Load Sequence Parameters.vi"("Reference values"=w226, "measurement configuration"=w229) -> ("load sequence parameters"=w227:T17)  [unwired: 9 in]
            n82 = call "Setup DCPower Current Sequence for ELOAD.vi"("error in (no error)"=w232, "Parameters for Sequence"=w227, "Channel List"=w228, "DCPower Handle In"=w233) -> ("error out"=w231:errorcluster, "DCPower Handle Out"=w225:refnum<k15>)  [unwired: 6 in]
            n83 = Bundle By Name(cluster=w226, "Load handle"=w225) -> (w224:T5)
            n84 = call "Configure Trigger for Load.vi"("error in (no error)"=w231, "Reference values"=w224) -> ("error out"=w235:errorcluster, "Reference values out"=w234:T5)  [unwired: 8 in]
          }
          frame "ConfigureAndInitiateScope" {
            w243 = TRUE  # Enable TClk
            n85 = Unbundle By Name(w237) -> ("Measure terminal name"=w241:string)
            n86 = Unbundle By Name(w238) -> ("Pin Names for Scope"=w242:string[])
            n87 = Bundle By Name(cluster=w237, "Enable TClk"=w243) -> (w244:T5)
            n88 = call "Create Scope Parameters.vi"("Reference values"=w237, "measurement configuration"=w238) -> ("scope parameters array"=w236:T7[])  [unwired: 9 in]
            n89 = case shown="True" w243 {
              tunnel: w247 -> [w261 w303]
              tunnel: w244 -> [w260 w297]
              tunnel: [w259 w291] -> w246
              tunnel: [w258 w298] -> w245
              tunnel: w236 -> [w251 w290]
              tunnel: w242 -> [w252 w288]
              tunnel: w241 -> [w250 w289]
              tunnel: w240 -> [w249 w287]
              tunnel: [w249 w287] -> w239
              frame False {
                # "TClk has not been supported by grpc-device and cannot be used with the Measurement Plug-In APIs as of 2024 Q4.\nFor strict synchronization with TClk, you need to use the niScope Initialize with Options VI to initialize sessions."
                n90 = Array Size(array=w252) -> (size(s)=w253:i32)
                n91 = case shown="1.." w253 {
                  tunnel: w249 -> [_ w273]
                  tunnel: w261 -> [w262 w272]
                  tunnel: w252 -> [_ w266]
                  tunnel: [_ w265] -> w257
                  tunnel: [w262 w264] -> w255
                  tunnel: [_ w263] -> w254
                  frame 0, Default {
                  }
                  frame 1.. {
                    n92 = call-poly <vilib>:"Reserve Sessions.vi"("error in"=w272, "pin or relay names"=w266, "measurement context in"=w273) -> ("error out"=w271:errorcluster, "session reservation out"=w270:refnum<class "Session Reservation.lvclass">)  [unwired: 6 in, 1 out]
                    n93 = call-poly <vilib>:"Initialize Sessions.vi"("error in"=w271, "reset"=FALSE, "session reservation in"=w270) -> ("error out"=w269:errorcluster, "session reservation out"=w268:refnum<class "Session Reservation.lvclass">)  [unwired: 5 in, 2 out]
                    n94 = call-poly <vilib>:"Get Connections.vi"("error in"=w269, "pin or relay names"=w266, "session reservation in"=w268) -> ("error out"=w264:errorcluster, "connections"=w263:T18[], "session reservation out"=w265:refnum<class "Session Reservation.lvclass">)  [unwired: 6 in]
                  }
                }
                n95 = for {
                  tunnel: w254 -> [w286] mode=indexing
                  shift-right: [w280] -> w256
                  shift-left: w255 -> [w283]
                  tunnel: w251 -> [w279] mode=indexing
                  tunnel: w250 -> [w278]
                  tunnel: [w277] -> w248 mode=indexing
                  n96 = Unbundle By Name(w286) -> ("session"=w285:refnum<k15>, "connection.channel"=w284:string)
                  n97 = call "Setup Scope.vi"("instrument handle"=w285, "channels"=w284, "Scope Parameters"=w279, "error in"=w283) -> ("instrument handle out"=w281:refnum<k15>, "error out"=w282:errorcluster)  [unwired: 10 in]
                  n98 = call-poly <instrlib>:"niScope Configure Trigger (poly).vi"("instrument handle"=w281, "trigger source"=w278, "error in"=w282) -> ("instrument handle out"=w277:refnum<k15>, "error out"=w280:errorcluster)  [unwired: 11 in]
                }
                n99 = for {
                  tunnel: w248 -> [w274] mode=indexing
                  shift-right: [w275] -> w258
                  shift-left: w256 -> [w276]
                  n100 = call <instrlib>:"niScope Initiate Acquisition.vi"("instrument handle"=w274, "error in"=w276) -> ("error out"=w275:errorcluster)  [unwired: 12 in, 1 out]
                }
                n101 = Bundle By Name(cluster=w260, "scope session reservation"=w257) -> (w259:T5)
              }
              frame True {
                n102 = call-dynamic "Get Pin Map Context.vi"("error in"=w303, "measure call context in"=w287) -> ("error out"=w301:errorcluster, "pin map context"=w302:T19)  [unwired: 7 in, 1 out]
                n103 = Unbundle By Name(w302) -> ("pin map id"=w300:string)
                n104 = Build Path(name or relative path=w300) -> (appended path=w299:path)  [unwired: 1 in]
                n105 = call "Create Connection Map From Pin Map File.vi"("error in (no error)"=w301, "pin map file path"=w299) -> ("error out"=w294:errorcluster, "connection map"=w296:map{string, T6[]})  [unwired: 8 in]
                n106 = call "Create Scope Info Map for Each Site.vi"("error in (no error)"=w294, "parameters array"=w290, "Pin Names for Scope"=w288, "connection map"=w296) -> ("error out"=w293:errorcluster, "scope info map for each site"=w295:T20)  [unwired: 6 in]
                n107 = for {
                  tunnel: w289 -> [w304]
                  shift-right: [w306] -> w298
                  shift-left: w293 -> [w307]
                  tunnel: [w305] -> w292 mode=indexing
                  tunnel: w295 -> [w308] mode=indexing
                  # "Loop for multiple sites"
                  n108 = call "Initialize Configure Initiate Scope with TClk.vi"("error in (no error)"=w307, "ref trigger source"=w304, "scope info map"=w308) -> ("error out"=w306:errorcluster, "scope handles"=w305:refnum<k15>[])  [unwired: 7 in]
                }
                n109 = Bundle By Name(cluster=w297, "connection map"=w296, "instrument info map array"=w295, "Scope handles"=w292) -> (w291:T5)
              }
            }
          }
          frame "ConfigureAndInitiateDMM" {
            n110 = Unbundle By Name(w314) -> ("dmm pin names"=w311:string[])
            n111 = Array Size(array=w311) -> (size(s)=w310:i32)
            n112 = Greater Than 0?(x=w310) -> (x > 0?=w309:bool)
            n113 = case shown="True" w309 {
              tunnel: w322 -> [w323 w333]
              tunnel: w321 -> [_ w332]
              tunnel: [_ w331] -> w320
              tunnel: [w323 w330] -> w319
              tunnel: w311 -> [_ w329]
              tunnel: [_ w328] -> w316
              frame False {
              }
              frame True {
                n114 = call-poly <vilib>:"Reserve Sessions.vi"("error in"=w333, "pin or relay names"=w329, "measurement context in"=w332) -> ("error out"=w327:errorcluster, "session reservation out"=w326:refnum<class "Session Reservation.lvclass">)  [unwired: 6 in, 1 out]
                n115 = call-poly <vilib>:"Initialize Sessions.vi"("error in"=w327, "session reservation in"=w326) -> ("error out"=w325:errorcluster, "session reservation out"=w324:refnum<class "Session Reservation.lvclass">)  [unwired: 6 in, 2 out]
                n116 = call-poly <vilib>:"Get Connections.vi"("error in"=w325, "pin or relay names"=w329, "session reservation in"=w324) -> ("error out"=w330:errorcluster, "connections"=w331:T21[], "session reservation out"=w328:refnum<class "Session Reservation.lvclass">)  [unwired: 6 in]
              }
            }
            n117 = call "Create DMM Parameters.vi"("Reference values"=w312, "measurement configuration"=w314) -> ("dmm parameters"=w313:T22[])  [unwired: 9 in]
            n118 = for {
              tunnel: w320 -> [w341] mode=indexing
              shift-right: [w340] -> w318
              shift-left: w319 -> [w337]
              tunnel: w313 -> [w335] mode=indexing
              tunnel: [w334] -> w317 mode=indexing
              n119 = Unbundle By Name(w341) -> ("session"=w336:refnum<k15>)
              n120 = call "Setup DMM to Acquire Multiple Samples.vi"("error in (no error)"=w337, "DMM Parameters"=w335, "instrument handle"=w336) -> ("error out"=w338:errorcluster, "instrument handle out"=w339:refnum<k15>)  [unwired: 7 in]
              n121 = call <instrlib>:"niDMM Initiate.vi"("error in (no error)"=w338, "instrument handle"=w339) -> ("error out"=w340:errorcluster, "instrument handle out"=w334:refnum<k15>)  [unwired: 8 in]
            }
            n122 = Bundle By Name(cluster=w312, "dmm session reservation"=w316, "dmm handle array"=w317) -> (w315:T5)
          }
          frame "StartSourceAndLoad" {
            n123 = call "Initiate Source And Load Sequence And Wait.vi"("error in (no error)"=w345, "Reference values"=w343) -> ("error out"=w344:errorcluster, "Reference values out"=w342:T5)  [unwired: 8 in]
          }
          frame "PerformMeasurement" {
            # "1.Fetches the voltages and currents of both the PPS and E-Load\n2.Calculates the efficiency (%), load voltage deviation (%)"
            n124 = call "Perform Measurements.vi"("Reference values"=w350, "measurement configuration"=w347, "Measurement Context"=w352, "error in"=w353) -> ("Reference values out"=w348:T5, "error out"=w351:errorcluster)  [unwired: 10 in]
            n125 = disable-structure shown="Enabled" {
              disable-tunnel: w351 -> [w357 w358]
              disable-tunnel: w348 -> [w356 _]
              disable-tunnel: [w355 w358] -> w349
              disable-tunnel: w347 -> [w354 _]
              frame Enabled {
                n126 = call "Save Results to TDMS.vi"("error in (no error)"=w357, "measurement configuration"=w354, "Reference values"=w356) -> ("error out"=w355:errorcluster)  [unwired: 8 in]
              }
              frame Disabled {
              }
            }
          }
          frame "Exit", Default {
            # "1. Aborts the channels\n2. Deletes the created advanced sequence\n3. Close all the opened sessions"
            n127 = Release Queue(queue=w362, error in (no error)=w367) -> (error out=w366:errorcluster)  [unwired: 1 in, 2 out]
            n128 = case shown="No Error" w366 {
              selector: w366 -> [w385 w441]
              tunnel: [w370 w432] -> w364
              tunnel: w365 -> [w388 w443]
              tunnel: [w394 w443] -> w363
              tunnel: w360 -> [w372 w436]
              frame No Error {
                # "Updates the status indicator on the operation performed if there is no error"
                n129 = Unbundle By Name(w388) -> ("Source handle array"=w377:refnum<k15>[], "Source channel name array"=w379:string[], "Source sequence name"=w393:string, "Load handle"=w383:refnum<k15>, "Load channel name"=w382:string)
                n130 = call <instrlib>:"niDCPower Configure Output Enabled.vi"("error in (no error)"=w385, "output enabled"=FALSE, "channel name"=w382, "instrument handle"=w383) -> ("error out"=w384:errorcluster, "instrument handle out"=w380:refnum<k15>)  [unwired: 6 in]
                n131 = call <instrlib>:"niDCPower Abort With Channels.vi"("error in (no error)"=w384, "channel name"=w382, "instrument handle"=w380) -> ("error out"=w378:errorcluster)  [unwired: 7 in, 1 out]
                n132 = for {
                  tunnel: w393 -> [w406]
                  tunnel: w379 -> [w404] mode=indexing
                  tunnel: w377 -> [w402] mode=indexing
                  shift-right: [w405] -> w391
                  shift-left: w378 -> [w403]
                  n133 = call <instrlib>:"niDCPower Abort With Channels.vi"("error in (no error)"=w403, "channel name"=w404, "instrument handle"=w402) -> ("error out"=w408:errorcluster, "instrument handle out"=w407:refnum<k15>)  [unwired: 7 in]
                  n134 = call <instrlib>:"niDCPower Delete Advanced Sequence With Channels.vi"("error in (no error)"=w408, "sequence name"=w406, "channel name"=w404, "instrument handle"=w407) -> ("error out"=w405:errorcluster)  [unwired: 6 in, 1 out]
                }
                n135 = Unbundle By Name(w388) -> ("dmm session reservation"=w369:refnum<class "Session Reservation.lvclass">, "Enable TClk"=w376:bool, "Scope handles"=w375:refnum<k15>[][], "scope session reservation"=w386:refnum<class "Session Reservation.lvclass">, "dcpower session reservation"=w387:refnum<class "Session Reservation.lvclass">)
                n136 = call <vilib>:"Close Sessions.vi"("error in"=w391, "session reservation in"=w387) -> ("error out"=w392:errorcluster, "session reservation out"=w390:refnum<class "Session Reservation.lvclass">)  [unwired: 8 in]
                n137 = call <vilib>:"Unreserve Sessions.vi"("error in"=w392, "session reservation in"=w390) -> ("error out"=w389:errorcluster)  [unwired: 9 in]
                n138 = case shown="False" w376 {
                  tunnel: w389 -> [w414 w422]
                  tunnel: [w413 w421] -> w371
                  tunnel: w386 -> [w412 _]
                  tunnel: w372 -> [w411 _]
                  tunnel: w375 -> [_ w423]
                  frame False {
                    n139 = Unbundle By Name(w411) -> ("Pin Names for Scope"=w410:string[])
                    n140 = Array Size(array=w410) -> (size(s)=w409:i32)
                    n141 = case shown="1.." w409 {
                      tunnel: w414 -> [w415 w419]
                      tunnel: [w415 w417] -> w413
                      tunnel: w412 -> [_ w416]
                      frame 0, Default {
                      }
                      frame 1.. {
                        n142 = call <vilib>:"Close Sessions.vi"("error in"=w419, "session reservation in"=w416) -> ("error out"=w418:errorcluster, "session reservation out"=w420:refnum<class "Session Reservation.lvclass">)  [unwired: 8 in]
                        n143 = call <vilib>:"Unreserve Sessions.vi"("error in"=w418, "session reservation in"=w420) -> ("error out"=w417:errorcluster)  [unwired: 9 in]
                      }
                    }
                  }
                  frame True {
                    n144 = for {
                      tunnel: w423 -> [w426] mode=indexing
                      shift-right: [w424] -> w421
                      shift-left: w422 -> [w425]
                      n145 = for {
                        tunnel: w426 -> [w427] mode=indexing
                        shift-right: [w428] -> w424
                        shift-left: w425 -> [w429]
                        n146 = call <instrlib>:"niScope Close.vi"("instrument handle"=w427, "error in"=w429) -> ("error out"=w428:errorcluster)  [unwired: 13 in]
                      }
                    }
                  }
                }
                n147 = Unbundle By Name(w372) -> ("dmm pin names"=w374:string[])
                n148 = Array Size(array=w374) -> (size(s)=w373:i32)
                n149 = Greater Than 0?(x=w373) -> (x > 0?=w368:bool)
                n150 = case shown="True" w368 {
                  tunnel: w371 -> [w396 w400]
                  tunnel: [w396 w399] -> w370
                  tunnel: w369 -> [_ w397]
                  frame False {
                  }
                  frame True {
                    n151 = call <vilib>:"Close Sessions.vi"("error in"=w400, "session reservation in"=w397) -> ("error out"=w401:errorcluster, "session reservation out"=w398:refnum<class "Session Reservation.lvclass">)  [unwired: 8 in]
                    n152 = call <vilib>:"Unreserve Sessions.vi"("error in"=w401, "session reservation in"=w398) -> ("error out"=w399:errorcluster)  [unwired: 9 in]
                  }
                }
                n153 = Bundle By Name(cluster=w388, "Measurement Results.Status"="The measurement is performed successfully" ("message")) -> (w394:T5)
              }
              frame Error {
                # "Resets the device with default values whenever there is an error"
                n154 = Unbundle By Name(w443) -> ("Source handle array"=w451:refnum<k15>[], "Source channel name array"=w449:string[], "Load handle"=w448:refnum<k15>, "Load channel name"=w447:string)
                n155 = call <instrlib>:"niDCPower Abort With Channels.vi"("error in (no error)"=w441, "channel name"=w447, "instrument handle"=w448) -> ("error out"=w453:errorcluster, "instrument handle out"=w452:refnum<k15>)  [unwired: 7 in]
                n156 = call <instrlib>:"niDCPower Reset With Channels.vi"("error in (no error)"=w453, "channel name"=w447, "instrument handle"=w452) -> ("error out"=w450:errorcluster)  [unwired: 7 in, 1 out]
                n157 = for {
                  tunnel: w451 -> [w463] mode=indexing
                  tunnel: w449 -> [w461] mode=indexing
                  shift-right: [w460] -> w445
                  shift-left: w450 -> [w462]
                  n158 = call <instrlib>:"niDCPower Abort With Channels.vi"("error in (no error)"=w462, "channel name"=w461, "instrument handle"=w463) -> ("error out"=w464:errorcluster, "instrument handle out"=w465:refnum<k15>)  [unwired: 7 in]
                  n159 = call <instrlib>:"niDCPower Reset With Channels.vi"("error in (no error)"=w464, "channel name"=w461, "instrument handle"=w465) -> ("error out"=w460:errorcluster)  [unwired: 7 in, 1 out]
                }
                n160 = Unbundle By Name(w443) -> ("dmm session reservation"=w430:refnum<class "Session Reservation.lvclass">, "Enable TClk"=w440:bool, "Scope handles"=w437:refnum<k15>[][], "scope session reservation"=w438:refnum<class "Session Reservation.lvclass">, "dcpower session reservation"=w442:refnum<class "Session Reservation.lvclass">)
                n161 = call <vilib>:"Close Sessions.vi"("error in"=w445, "session reservation in"=w442) -> ("error out"=w446:errorcluster, "session reservation out"=w444:refnum<class "Session Reservation.lvclass">)  [unwired: 8 in]
                n162 = call <vilib>:"Unreserve Sessions.vi"("error in"=w446, "session reservation in"=w444) -> ("error out"=w439:errorcluster)  [unwired: 9 in]
                n163 = case shown="False" w440 {
                  tunnel: w439 -> [w471 w479]
                  tunnel: [w470 w478] -> w433
                  tunnel: w438 -> [w469 _]
                  tunnel: w436 -> [w468 _]
                  tunnel: w437 -> [_ w480]
                  frame False {
                    n164 = Unbundle By Name(w468) -> ("Pin Names for Scope"=w467:string[])
                    n165 = Array Size(array=w467) -> (size(s)=w466:i32)
                    n166 = case shown="1.." w466 {
                      tunnel: w471 -> [w472 w476]
                      tunnel: [w472 w474] -> w470
                      tunnel: w469 -> [_ w473]
                      frame 0, Default {
                      }
                      frame 1.. {
                        n167 = call <vilib>:"Close Sessions.vi"("error in"=w476, "session reservation in"=w473) -> ("error out"=w475:errorcluster, "session reservation out"=w477:refnum<class "Session Reservation.lvclass">)  [unwired: 8 in]
                        n168 = call <vilib>:"Unreserve Sessions.vi"("error in"=w475, "session reservation in"=w477) -> ("error out"=w474:errorcluster)  [unwired: 9 in]
                      }
                    }
                  }
                  frame True {
                    n169 = for {
                      tunnel: w480 -> [w483] mode=indexing
                      shift-right: [w481] -> w478
                      shift-left: w479 -> [w482]
                      n170 = for {
                        tunnel: w483 -> [w484] mode=indexing
                        shift-right: [w485] -> w481
                        shift-left: w482 -> [w486]
                        n171 = call <instrlib>:"niScope Close.vi"("instrument handle"=w484, "error in"=w486) -> ("error out"=w485:errorcluster)  [unwired: 13 in]
                      }
                    }
                  }
                }
                n172 = Unbundle By Name(w436) -> ("dmm pin names"=w435:string[])
                n173 = Array Size(array=w435) -> (size(s)=w434:i32)
                n174 = Greater Than 0?(x=w434) -> (x > 0?=w431:bool)
                n175 = case shown="True" w431 {
                  tunnel: w433 -> [w454 w458]
                  tunnel: [w454 w457] -> w432
                  tunnel: w430 -> [_ w455]
                  frame False {
                  }
                  frame True {
                    n176 = call <vilib>:"Close Sessions.vi"("error in"=w458, "session reservation in"=w455) -> ("error out"=w459:errorcluster, "session reservation out"=w456:refnum<class "Session Reservation.lvclass">)  [unwired: 8 in]
                    n177 = call <vilib>:"Unreserve Sessions.vi"("error in"=w459, "session reservation in"=w456) -> ("error out"=w457:errorcluster)  [unwired: 9 in]
                  }
                }
              }
            }
          }
        }
      }
    }
    frame "Power off the DUT" {
      # "Stops generation on the output channel and resets the channels to default values"
      n178 = Unbundle By Name(w530) -> ("Source pin name array"=w501:string[], "Load pin name"=w507:string)
      n179 = Build Array (concatenate)(w501, w507) -> (w522:string[])
      n180 = call-poly <vilib>:"Reserve Sessions.vi"("timeout (ms)"=60000, "error in"=w521, "pin or relay names"=w522, "measurement context in"=w519) -> ("error out"=w526:errorcluster, "session reservation out"=w525:refnum<class "Session Reservation.lvclass">)  [unwired: 5 in, 1 out]
      n181 = call-poly <vilib>:"Initialize Sessions.vi"("error in"=w526, "session reservation in"=w525) -> ("error out"=w524:errorcluster, "session reservation out"=w523:refnum<class "Session Reservation.lvclass">)  [unwired: 6 in, 2 out]
      n182 = call-poly <vilib>:"Get Connections.vi"("error in"=w524, "pin or relay name"=w507, "session reservation in"=w523) -> ("error out"=w514:errorcluster, "connection"=w518:T14, "session reservation out"=w508:refnum<class "Session Reservation.lvclass">)  [unwired: 6 in]
      n183 = Unbundle By Name(w518) -> ("session"=w513:refnum<k15>, "connection.channel"=w512:string)
      n184 = call <instrlib>:"niDCPower Configure Output Enabled.vi"("error in (no error)"=w514, "output enabled"=FALSE, "channel name"=w512, "instrument handle"=w513) -> ("error out"=w515:errorcluster, "instrument handle out"=w516:refnum<k15>)  [unwired: 6 in]
      n185 = call <instrlib>:"niDCPower Reset With Channels.vi"("error in (no error)"=w515, "channel name"=w512, "instrument handle"=w516) -> ("error out"=w509:errorcluster)  [unwired: 7 in, 1 out]
      n186 = call-poly <vilib>:"Get Connections.vi"("error in"=w509, "pin or relay names"=w501, "session reservation in"=w508) -> ("error out"=w511:errorcluster, "connections"=w510:T14[], "session reservation out"=w504:refnum<class "Session Reservation.lvclass">)  [unwired: 6 in]
      n187 = for {
        tunnel: w510 -> [w532] mode=indexing
        shift-right: [w531] -> w506
        shift-left: w511 -> [w536]
        n188 = Unbundle By Name(w532) -> ("session"=w537:refnum<k15>, "connection.channel"=w538:string)
        n189 = call <instrlib>:"niDCPower Configure Output Enabled.vi"("error in (no error)"=w536, "output enabled"=FALSE, "channel name"=w538, "instrument handle"=w537) -> ("error out"=w535:errorcluster, "instrument handle out"=w534:refnum<k15>)  [unwired: 6 in]
        n190 = call <instrlib>:"niDCPower Reset With Channels.vi"("error in (no error)"=w535, "channel name"=w538, "instrument handle"=w534) -> ("error out"=w531:errorcluster)  [unwired: 7 in, 1 out]
      }
      n191 = call <vilib>:"Close Sessions.vi"("error in"=w506, "session reservation in"=w504) -> ("error out"=w505:errorcluster, "session reservation out"=w503:refnum<class "Session Reservation.lvclass">)  [unwired: 8 in]
      n192 = call <vilib>:"Unreserve Sessions.vi"("error in"=w505, "session reservation in"=w503) -> ("error out"=w502:errorcluster)  [unwired: 9 in]
      n193 = Bundle By Name(cluster=w529, "Measurement Results.Status"="The DUT is powered OFF") -> (w527:T5)
    }
  }
  "error out" <- w6
  "measure call context out" <- w8
  n194 = Unbundle By Name(w7) -> ("Measurement Results"=→"measurement results":T1)
